vi "NavX Heading.vi"(8 "error in":errorcluster) -> (0 "error out":errorcluster, 2 "Absolute Heading":dbl, 3 "Heading":dbl)   [LabVIEW 2015]
uses:
  Support/Global Objects.vi
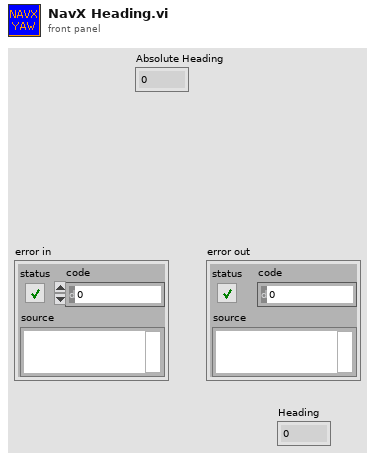
[diagram p1: front panel]
types:
  T1 = typedef "NaxX Info.ctl" = cluster{"navX Device":T2, "Current Yaw":dbl, "Active":bool}
  T2 = typedef "navX Library v2.lvlib/Z900_navX_DeviceTypeDef.ctl" = cluster{"Interface":cluster{"Protocol":T3, "Update Rate (4Hz-60Hz)":u8, "navX Open TypeDef":variant}, "Notify Packet":refnum<notifier>, "Loop VI Refnum":refnum<vi>, "Ready to Close Occurrence Refnum":refnum<k4>}
  T3 = typedef "navX Library v2.lvlib/Z900_navX_ProtocolTypeDef.ctl" = enum16{"SERIAL", "I2C", "SPI"}
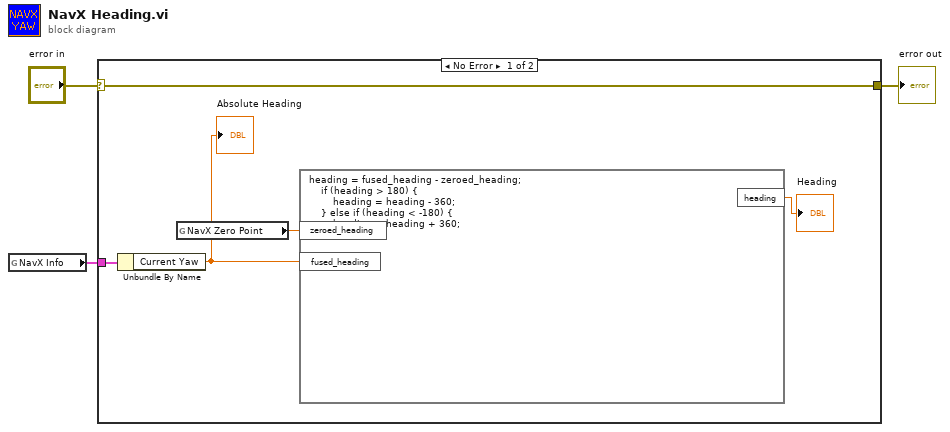
[diagram p0: block diagram]
diagram:
  n1 = global read "Global Objects.vi" "NavX Info"() -> (w1:T1)
  n2 = case shown="No Error" "error in" {
    selector: "error in" -> [w7 w9]
    tunnel: [w7 w9] -> w2
    tunnel: w1 -> [w4 _]
    frame No Error {
      n3 = Unbundle By Name(w4) -> ("Current Yaw"=w6:dbl)
      "Absolute Heading" <- w6
      n4 = global read "Global Objects.vi" "NavX Zero Point"() -> (w5:dbl)
      n5 = formula code="heading = fused_heading - zeroed_heading;\n    if (heading > 180) {\n        heading = heading - 360;\n    } else if (heading < -180) {\n        heading = heading + 360;\n    }"("zeroed_heading"=w5, "fused_heading"=w6) -> ("heading"=→"Heading":dbl)
    }
    frame Error {
    }
  }
  "error out" <- w2
